vi "Sub_Preprocessing_FEA_and_LEMP.vi"(2 "Modeling Parameters":T1, 3 "FEA Parameters":T2={"LEMP"={"Eigenvalues"=[], "Square Transpose Eigenvectors"=[], "1/deltaStiff"=0.0}, "nodes of interest"=[], "all nodes"=[], "Eigenvalue Method"=enum."0-Local Eigen Modification Procedure", "Mode Count"=3, "initial_pin_node"=0, "Sub Sample"=TRUE}) -> (0 "Modeling Parameters":T1, 1 "FEA Parameters":T2={"LEMP"={"Eigenvalues"=[], "Square Transpose Eigenvectors"=[], "1/deltaStiff"=0.0}, "nodes of interest"=[], "all nodes"=[], "Eigenvalue Method"=enum."0-Local Eigen Modification Procedure", "Mode Count"=3, "initial_pin_node"=0, "Sub Sample"=TRUE})   [LabVIEW 2021]
panel:
  # "Input"
  # "Output"
  # "This VI acquires the required input cluster for the Sub_online_LEMP_Update.vi, this VI calls on SciPy.linalg.eigh() due to issues with the standard \"General Eigenvalues and Eigenvectors.vi\" outputting inappropriately scaled eigenvectors for the LEMP. Additionally the Bitedness of this installation of LabVIEW does not match with Python so direct python calls were similarly unavailable. The workaround involved a saving the matrices in a text format command line calling the SciPy eigh function saving that output as a text file, then load the output file in to memory (See Sub_Python_cmd_eigh.vi, getEigenCommandPrompt.py , mass.lvm, stiff.lvm,eigenvalues.txt, eigenvectors.txt).\n\n              - Alexander Vereen AFRL Summer scholars 2022"
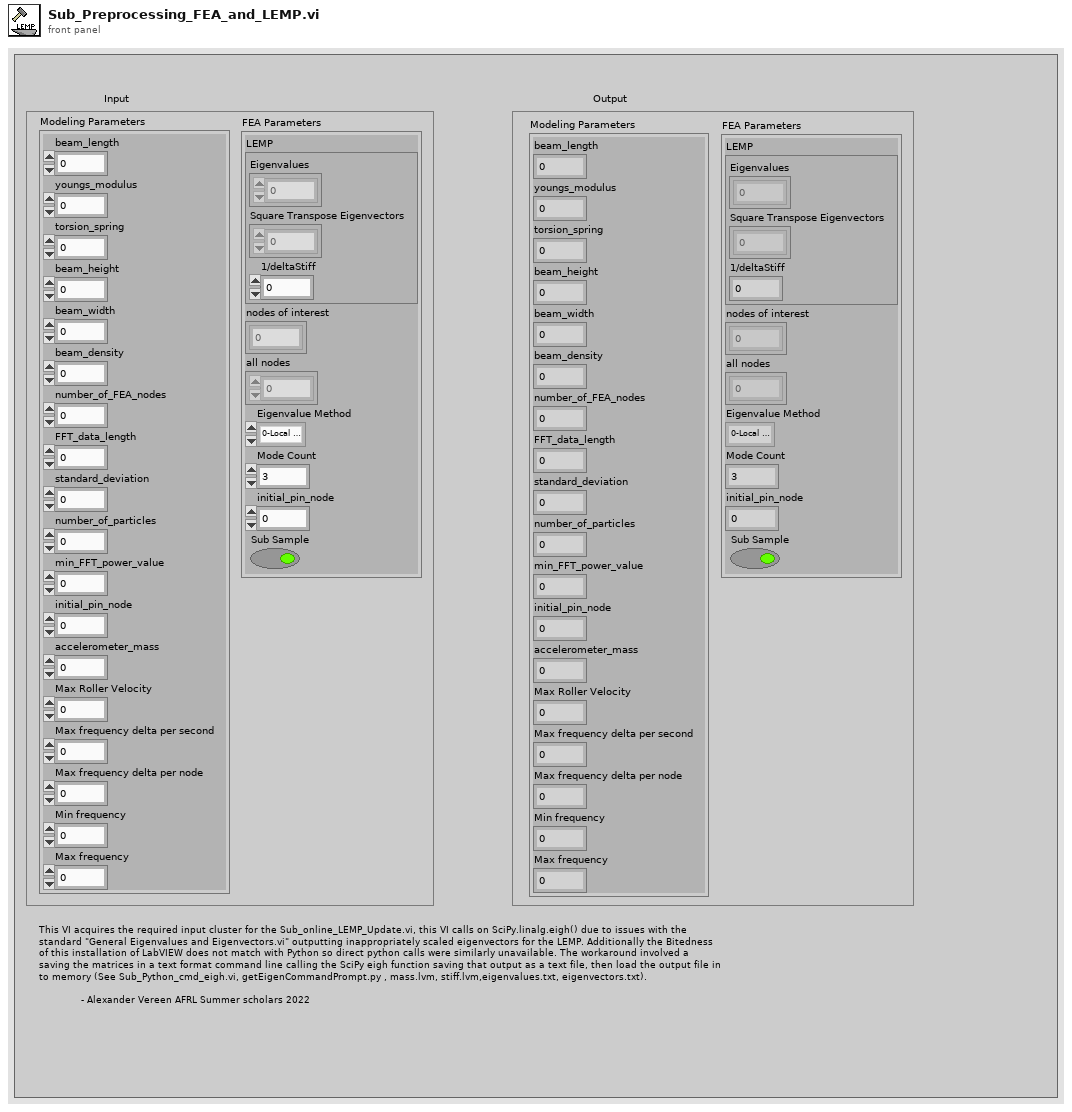
[diagram p1: front panel]
types:
  T1 = cluster{"beam_length":dbl, "youngs_modulus":dbl, "torsion_spring":dbl, "beam_height":dbl, "beam_width":dbl, "beam_density":dbl, "number_of_FEA_nodes":i32, "FFT_data_length":i32, "standard_deviation":dbl, "number_of_particles":i32, "min_FFT_power_value":dbl, "initial_pin_node":i32, "accelerometer_mass":dbl, "Max Roller Velocity":dbl, "Max frequency delta per second":dbl, "Max frequency delta per node":dbl, "Min frequency":dbl, "Max frequency":dbl}
  T2 = cluster{"LEMP":cluster{"Eigenvalues":dbl[], "Square Transpose Eigenvectors":dbl[][], "1/deltaStiff":dbl}, "nodes of interest":i32[], "all nodes":i32[], "Eigenvalue Method":enum16{"0-Local Eigen Modification Procedure", "1-LabVIEW generalized eigenvalues", "2-LabVIEW M^-1K eigenvalues", "3-LabVIEW Cholesky Factorization", "4-Cholesky Factorization CPU SGL", "5-Cholesky Factorization CPU FXP", "6-Cholesky Factorization FPGA SGL", "7-Cholesky Factorization FPGA SGL SCL"}, "Mode Count":i32, "initial_pin_node":i32, "Sub Sample":bool}
  T3 = cluster{"Eigenvalues":dbl[], "Square Transpose Eigenvectors":dbl[][], "1/deltaStiff":dbl}
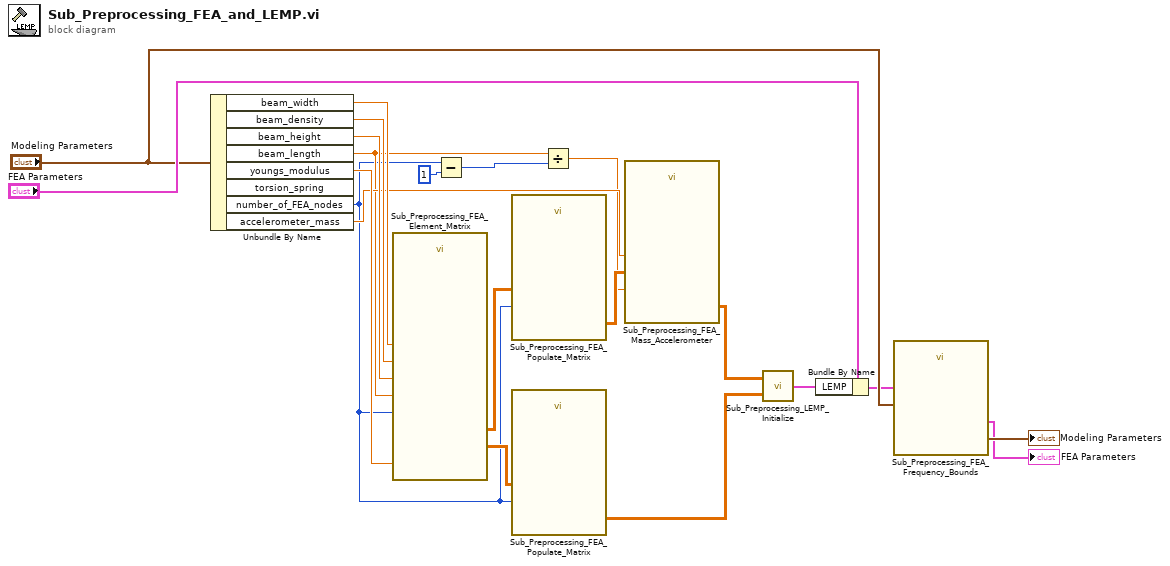
[diagram p0: block diagram]
diagram:
  n1 = Unbundle By Name("Modeling Parameters") -> ("beam_width"=w16:dbl, "beam_density"=w17:dbl, "beam_height"=w18:dbl, "beam_length"=w11:dbl, "youngs_modulus"=w19:dbl, "number_of_FEA_nodes"=w9:i32, "accelerometer_mass"=w12:dbl)  [unwired: 1 out]
  n2 = call "Sub_Preprocessing_FEA_Element_Matrix.vi"("Length of Beam"=w11, "Young's Modulus"=w19, "No. of Nodes"=w9, "Height"=w18, "Width"=w16, "Density"=w17) -> ("M Element Matrix"=w20:dbl[][], "K Element Matrix"=w21:dbl[][])  [unwired: 11 in, 1 out]
  n3 = Subtract(x=w9, y=1) -> (x-y=w14:i32)
  n4 = call "Sub_Preprocessing_FEA_Populate_Matrix.vi"("No. of Nodes"=w9, "Element Matrix"=w20) -> ("Matrix w/o BC"=w15:dbl[][])  [unwired: 9 in]
  n5 = call "Sub_Preprocessing_FEA_Populate_Matrix.vi"("No. of Nodes"=w9, "Element Matrix"=w21) -> ("Matrix w/o BC"=w7:dbl[][])  [unwired: 9 in]
  n6 = Divide(x=w11, y=w14) -> (x/y=w10:dbl)
  n7 = call "Sub_Preprocessing_FEA_Mass_Accelerometer.vi"("Element Length"=w15, "accelerometer_mass"=w12, "Matrix w/o BC"=w10) -> ("Matrix W/ Accelerometer"=w8:dbl[][])  [unwired: 8 in]
  n8 = call "Sub_Preprocessing_LEMP_Initialize.vi"("Stiff"=w7, "Mass"=w8) -> ("LEMP"=w5:T3)
  n9 = Bundle By Name(cluster="FEA Parameters", "LEMP"=w5) -> (w3:T2)
  n10 = call "Sub_Preprocessing_FEA_Frequency_Bounds.vi"("FEA Parameters"=w3, "Modeling Parameters"="Modeling Parameters") -> ("FEA Parameters"=→"FEA Parameters":T2, "Modeling Parameters"=→"Modeling Parameters":T1)
